vi "SECoP-showGUI.vi"(8 "error in (no error)":errorcluster, 10 "show GUI":bool=TRUE, 11 "DLL path (in)":T1) -> (0 "error out":errorcluster, 3 "DLL path (out)":T1)   [LabVIEW 2023, in "SECoP.lvlib"]
doc: "Call <b>\"SECoP-showGUI.vi\"</b> to show or hide the SHALL status window.\n\n<b>DLL path</b> input and output of cluster from \"SECoP-Initialize.vi\"\n<b>show status window (GUI)</b> boolean value to <b>show</b> (true) or <b>hide</b> (false) the status window"
uses:
  SECoP.lvlib
  SECoP-libraries.ctl
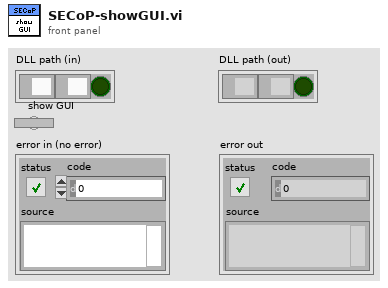
[diagram p1: front panel]
types:
  T1 = typedef "SECoP.lvlib/SECoP-libraries.ctl" = cluster{"serverDLL":path, "variantDLL":path, "cleanup_mode":bool}
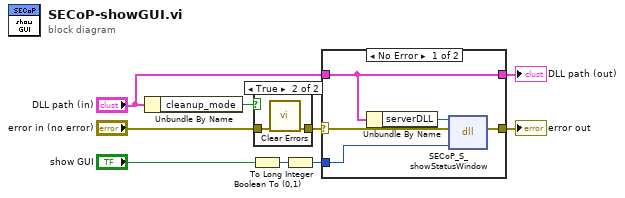
[diagram p0: block diagram]
diagram:
  n1 = Unbundle By Name("DLL path (in)") -> ("cleanup_mode"=w9:bool)
  n2 = Boolean To (0,1)(Boolean="show GUI") -> (0, 1=w4:i16)
  n3 = case shown="True" w9 {
    tunnel: "error in (no error)" -> [w10 w12]
    tunnel: [w10 w11] -> w8
    frame False {
    }
    frame True {
      n4 = call <vilib>:"Clear Errors.vi"("error in (no error)"=w12) -> ("error out"=w11:errorcluster)  [unwired: 5 in, 1 out]
    }
  }
  n5 = To Long Integer(number=w4) -> (32bit integer=w3:i32)
  n6 = case shown="No Error" w8 {
    selector: w8 -> [w17 w18]
    tunnel: "DLL path (in)" -> [w14 w19]
    tunnel: [w14 w19] -> w1
    tunnel: [w15 w18] -> w2
    tunnel: w3 -> [w16 _]
    frame No Error {
      n7 = Unbundle By Name(w14) -> ("serverDLL"=w13:path)
      n8 = dll-call lib="C:/Users/user/Desktop/x86_64/SECoP64.dll" fn="SECoP_S_showStatusWindow"(path in=w13, error in=w17, "bShowGUI"=w16) -> (error out=w15:errorcluster)  [unwired: 3 in, 1 out]
    }
    frame Error {
    }
  }
  "DLL path (out)" <- w1
  "error out" <- w2
